vi "Set Program State.vi"(8 "error in (no error)":errorcluster, 10 "Program Prameter":T3, 11 "Abstract in":refnum<class "Abstract.lvclass">) -> (0 "error out":errorcluster, 2 "Status":cluster{"ACK":bool, "Error":bool, "NACK":bool}, 3 "Abstract out":refnum<class "Abstract.lvclass">)   [LabVIEW 2021, in "Environment Chamber.lvlib" / "Abstract.lvclass"]
uses:
  Abstract.lvclass
  Support Libraries/Climatic Chamber/Private/Type Defs/Program CtrlState Enum.ctl
  Support Libraries/Climatic Chamber/Private/Type Defs/Program CtrlEndCond Enum.ctl
  Support Libraries/Climatic Chamber/Climatic Chamber.lvlib
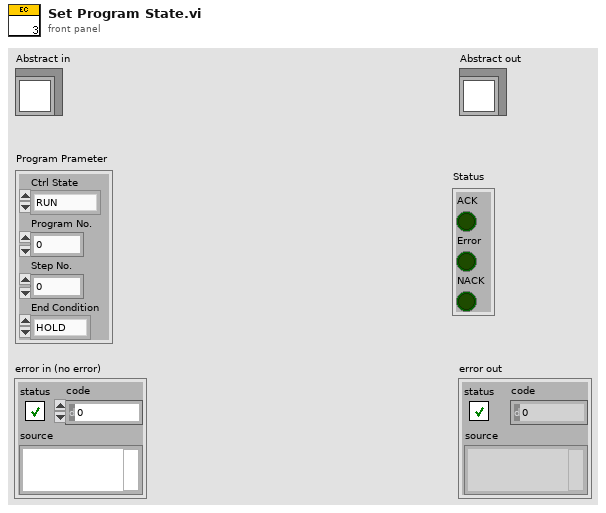
[diagram p1: front panel]
types:
  T1 = typedef "Environment Chamber.lvlib/Climatic Chamber.lvlib/Program CtrlState Enum.ctl" = enum16{"RUN", "PAUSE", "CONTINUE", "ADVANCE", "END"}
  T2 = typedef "Environment Chamber.lvlib/Climatic Chamber.lvlib/Program CtrlEndCond Enum.ctl" = enum16{"HOLD", "CONST", "OFF", "STANDBY"}
  T3 = cluster{"Ctrl State":T1, "Program No.":i32, "Step No.":i32, "End Condition":T2}
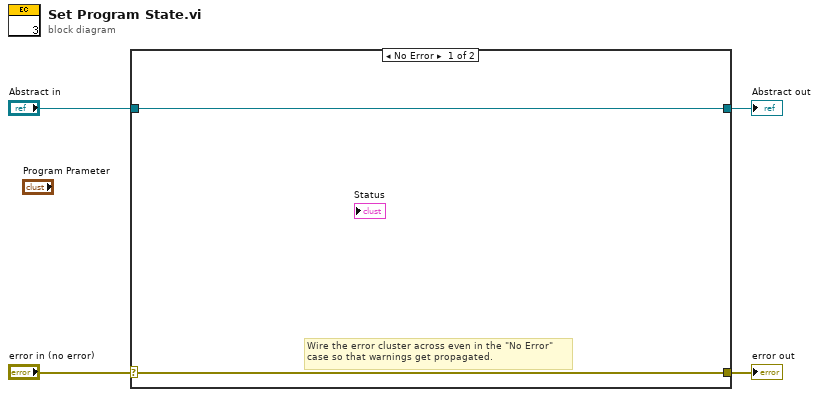
[diagram p0: block diagram]
diagram:
  n1 = case shown="No Error" "error in (no error)" {
    selector: "error in (no error)" -> [w5 w8]
    tunnel: [w5 w8] -> w3
    tunnel: [w6 w7] -> w1
    tunnel: "Abstract in" -> [w6 w7]
    frame No Error {
      # "Wire the error cluster across even in the \"No Error\"\ncase so that warnings get propagated."
    }
    frame Error {
    }
  }
  "error out" <- w3
  "Abstract out" <- w1
